vi "Handle Command.vi"(8 "error in (no error)":errorcluster, 9 "Data":variant, 10 "Command":string, 11 "Instrument.Oxford1820 in":refnum<class "Instrument.OxfordVRM.lvclass">) -> (0 "error out":errorcluster, 1 "Processed Data":variant, 2 "Command":string, 3 "Instrument.Oxford1820 out":refnum<class "Instrument.OxfordVRM.lvclass">)   [LabVIEW 2016, in "Instrument.OxfordVRM.lvclass"]
uses:
  Instrument.OxfordVRM.lvclass
  Typedefs/Instrument.Oxford1820.Commands-enum.ctl
  <instrlib>/Mercury iXX/Public/Libraries/Magnet/Controls/PSU Actions.ctl
  Typedefs/Targets.ctl
  Typedefs/PrivateEvents--Instrument.Oxford1820.SequenceSetMagnetField.ctl
  Typedefs/Instrument.Oxford1820.setMagnet-cluster.ctl
  <instrlib>/Mercury iXX/Public/Libraries/Magnet/Controls/Switch Heater.ctl
  Typedefs/Fill Mode-Combo.ctl
  <userlib>/LevyLab/Levylab Instruments/Instrument Types/Cryostat/Instrument.Cryostat.lvclass
  <instrlib>/Mercury iXX/Public/Libraries/Magnet.lvlib
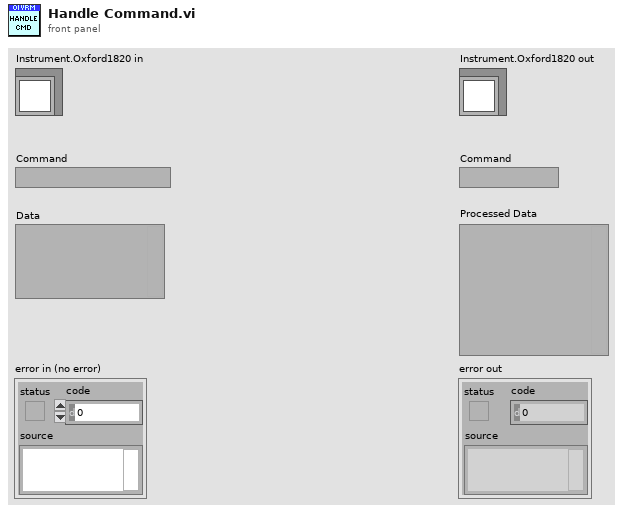
[diagram p1: front panel]
types:
  T1 = typedef "Instrument.OxfordVRM.lvclass/Instrument.Oxford1820.Commands-enum.ctl" = enum16{"setAction", "setTarget", "setSwitchHeat", "setLambda", "setFillMode", "setNeedleValve", "setMagnetField", "getStatus", "getTarget", "getSwitchHeat", "getPSUField", "newcommand", "getMagnetField"}
  T2 = typedef "Mercury iXX.lvlib/Magnet.lvlib/PSU Actions.ctl" = string
  T3 = typedef "Instrument.OxfordVRM.lvclass/Targets.ctl" = cluster{"Field (T)":dbl, "Field Rate (T/min)":dbl}
  T4 = typedef "Instrument.OxfordVRM.lvclass/Instrument.Oxford1820.setMagnet-cluster.ctl" = cluster{"Target":T3, "persistent mode":bool}
  T5 = typedef "Instrument.OxfordVRM.lvclass/PrivateEvents--Instrument.Oxford1820.SequenceSetMagnetField.ctl" = cluster{"setMagnet":T4}
  T6 = typedef "Mercury iXX.lvlib/Magnet.lvlib/Switch Heater.ctl" = string
  T7 = typedef "Instrument.OxfordVRM.lvclass/Fill Mode-Combo.ctl" = string
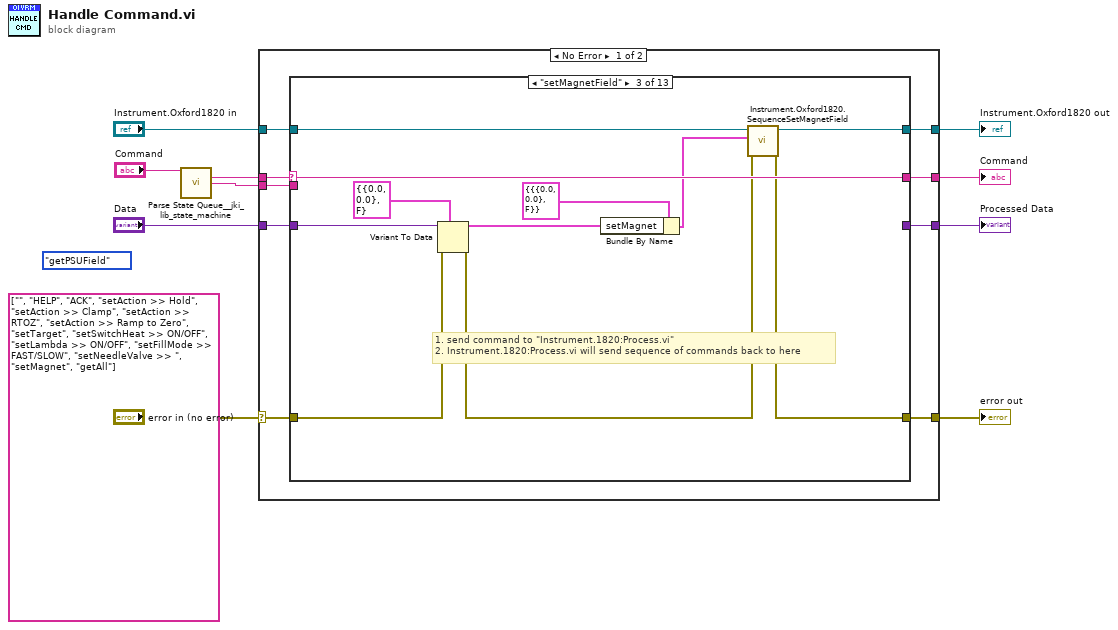
[diagram p0: block diagram]
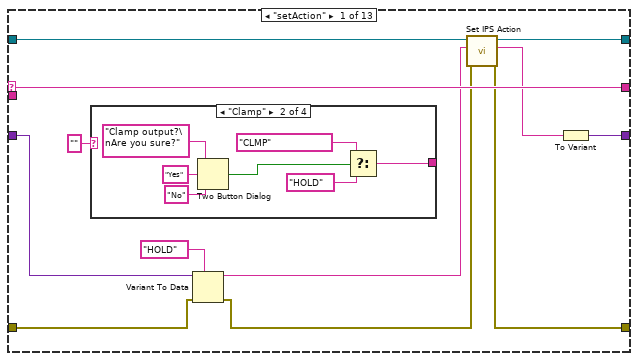
[diagram p2: hidden frame]
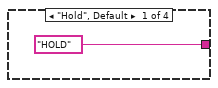
[diagram p3: hidden frame]
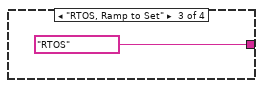
[diagram p4: hidden frame]
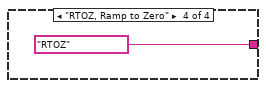
[diagram p5: hidden frame]
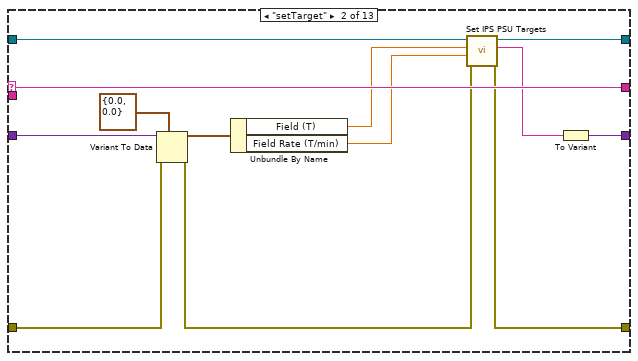
[diagram p6: hidden frame]
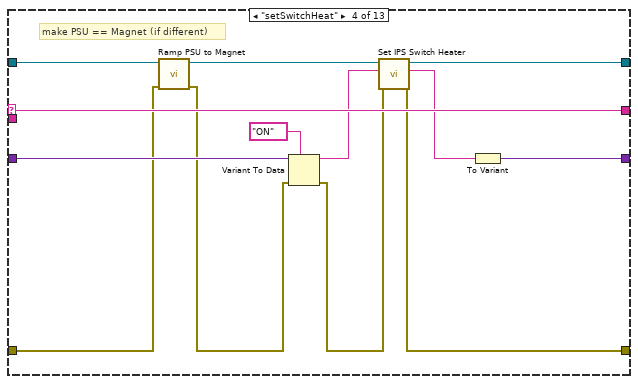
[diagram p7: hidden frame]
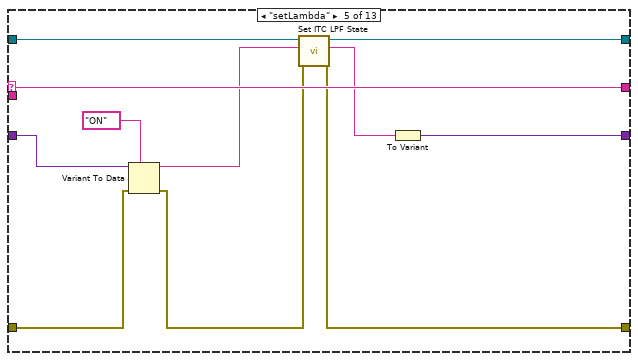
[diagram p8: hidden frame]
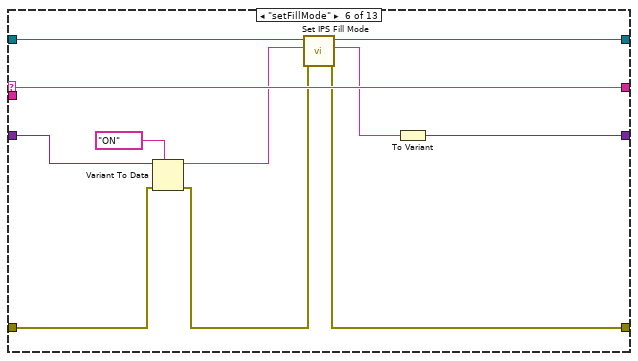
[diagram p9: hidden frame]
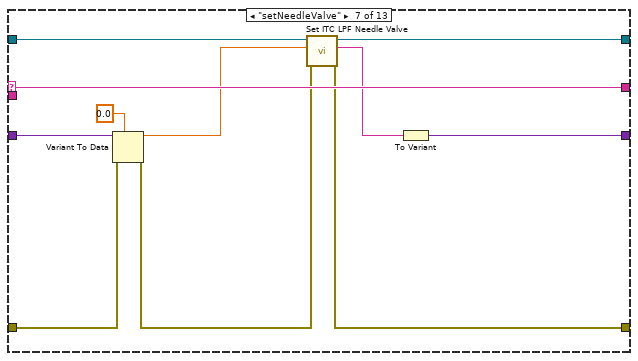
[diagram p10: hidden frame]
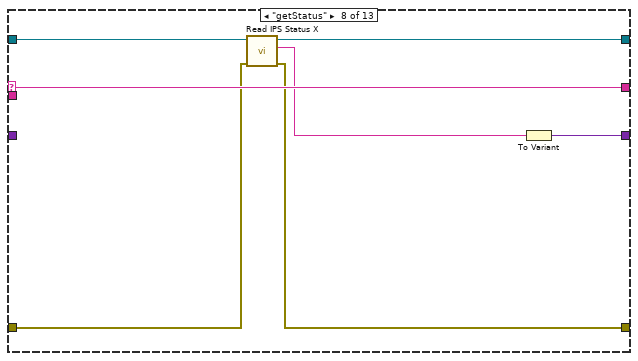
[diagram p11: hidden frame]
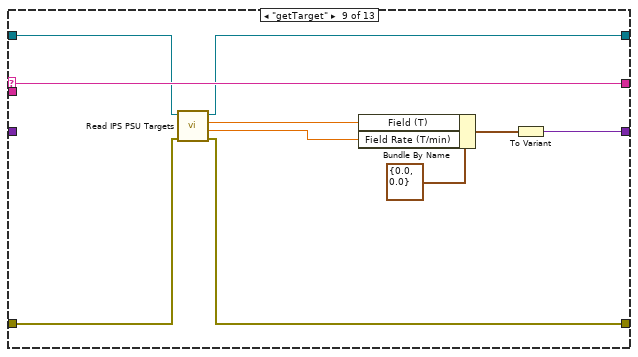
[diagram p12: hidden frame]
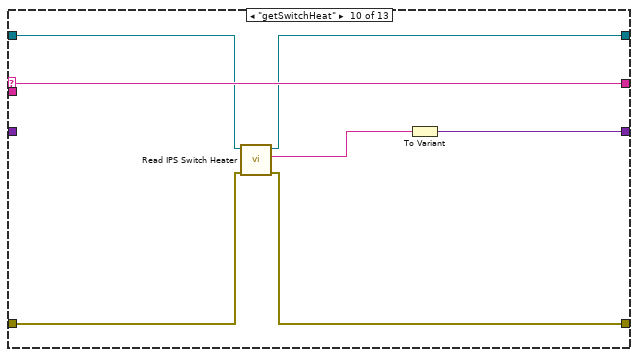
[diagram p13: hidden frame]
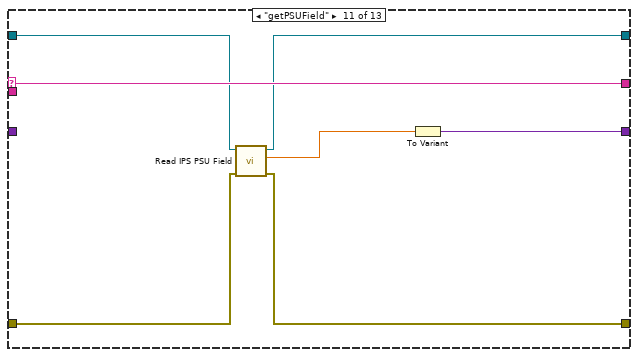
[diagram p14: hidden frame]
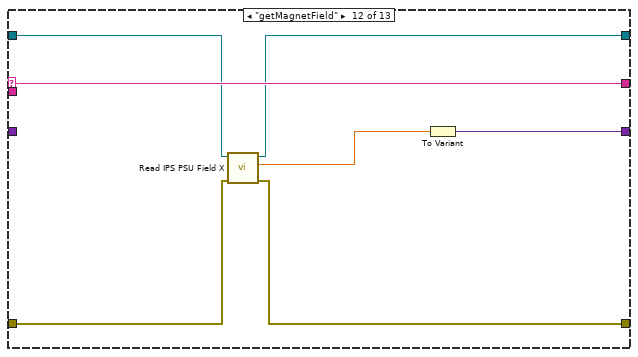
[diagram p15: hidden frame]
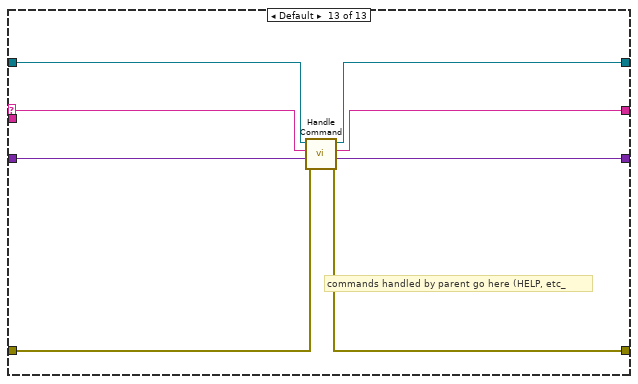
[diagram p16: hidden frame]
diagram:
  (unwired) Instrument.Oxford1820.Commands-enum."getPSUField" ("Commands")
  (unwired) string[] ["", "HELP", "ACK", "setAction >> Hold", "setAction >> Clamp", "setAction >> RTOZ", "setAction >> Ramp to Zero", "setTarget", "setSwitchHeat >> ON/OFF", "setLambda >> ON/OFF", "setFillMode >> FAST/SLOW", "setNeedleValve >> ", "setMagnet", "getAll"] ("Commands")
  n1 = call <vilib>:"Parse State Queue__jki_lib_state_machine.vi"("State Queue"="Command") -> ("Current State"=w2:string, "Arguments"=w1:string)  [unwired: 12 in, 1 out]
  n2 = case shown="No Error" "error in (no error)" {
    selector: "error in (no error)" -> [w14 w158]
    tunnel: [w13 w158] -> w10
    tunnel: [w19 _] -> w9
    tunnel: [w18 _] -> w8
    tunnel: [w17 w159] -> w7
    tunnel: "Data" -> [w16 _]
    tunnel: w2 -> [w11 _]
    tunnel: "Instrument.Oxford1820 in" -> [w15 w159]
    tunnel: w1 -> [w12 _]
    frame No Error {
      n3 = case shown="\"setMagnetField\"" w11 {
        selector: w11 -> [w31 w54 w65 w78 w89 w100 w111 w118 w128 w135 w142 w149 w150]
        tunnel: [w26 w49 _ w74 w84 w95 w106 w117 w127 w134 w141 w148 w157] -> w19
        tunnel: [w31 w54 w65 w78 w89 w100 w111 w118 w128 w135 w142 w149 w156] -> w18
        tunnel: [w29 w52 w63 w77 w87 w98 w109 w112 w120 w132 w139 w147 w155] -> w17
        tunnel: w16 -> [w25 w48 w61 w71 w82 w94 w104 _ _ _ _ _ w154]
        tunnel: w15 -> [w30 w53 w64 w73 w88 w99 w110 w113 w119 w133 w140 w143 w153]
        tunnel: w14 -> [w23 w43 w60 w69 w81 w92 w102 w116 w122 w131 w138 w145 w152]
        tunnel: [w28 w51 w62 w76 w86 w97 w108 w115 w121 w130 w137 w144 w151] -> w13
        tunnel: w12 -> [_ _ _ _ _ _ _ _ _ _ _ _ _]
        frame "setAction" {
          n4 = case shown="\"Clamp\"" "" {
            tunnel: [T2 "HOLD" ("PSU Act Stat") w38 T2 "RTOS" ("PSU Act Stat") T2 "RTOZ" ("PSU Act Stat")] -> _
            frame "Hold", Default {
            }
            frame "Clamp" {
              n5 = Two Button Dialog(message="Clamp output?\nAre you sure?", 1:"No" ("F button name (\"Cancel\")"), 2:"Yes" ("T button name (\"OK\")")) -> (T button?=w37:bool)
              n6 = Select(t=T2 "CLMP" ("PSU Act Stat"), s=w37, f=T2 "HOLD" ("PSU Act Stat")) -> (s? t:f=w38:T2)
            }
            frame "RTOS, Ramp to Set" {
            }
            frame "RTOZ, Ramp to Zero" {
            }
          }
          n7 = Variant To Data(error in=w23, type=T2 "HOLD" ("PSU Act Stat"), Variant=w25) -> (data=w21:T2, error out=w22:errorcluster)
          n8 = call "Set IPS Action.vi"("error in (no error)"=w22, "PSU Act Stat"=w21, "Instrument.OxfordVRM in"=w30) -> ("error out"=w28:errorcluster, "Response"=w27:string, "Instrument.OxfordVRM out"=w29:refnum<class "Instrument.OxfordVRM.lvclass">)  [unwired: 6 in]
          n9 = To Variant(anything=w27) -> (Variant=w26:variant)
        }
        frame "setTarget" {
          n10 = Variant To Data(error in=w43, type=T3 {"Field (T)"=0.0, "Field Rate (T/min)"=0.0} ("Targets"), Variant=w48) -> (data=w46:T3, error out=w42:errorcluster)
          n11 = Unbundle By Name(w46) -> ("Field (T)"=w45:dbl, "Field Rate (T/min)"=w44:dbl)
          n12 = call "Set IPS PSU Targets.vi"("error in (no error)"=w42, "Target Field Rate (T/min)"=w44, "Target Field (T)"=w45, "Instrument.OxfordVRM in"=w53) -> ("error out"=w51:errorcluster, "Response"=w50:string, "Instrument.OxfordVRM out"=w52:refnum<class "Instrument.OxfordVRM.lvclass">)  [unwired: 5 in]
          n13 = To Variant(anything=w50) -> (Variant=w49:variant)
        }
        frame "setMagnetField" {
          # "1. send command to \"Instrument.1820:Process.vi\"\n2. Instrument.1820:Process.vi will send sequence of commands back to here"
          n14 = Variant To Data(error in=w60, type=T4 {"Target"={"Field (T)"=0.0, "Field Rate (T/min)"=0.0}, "persistent mode"=FALSE} ("output cluster"), Variant=w61) -> (data=w56:T4, error out=w59:errorcluster)
          n15 = Bundle By Name(cluster=T5 {"setMagnet"={"Target"={"Field (T)"=0.0, "Field Rate (T/min)"=0.0}, "persistent mode"=FALSE}} ("Set Magnet Field"), "setMagnet"=w56) -> (w58:T5)
          n16 = call "Instrument.Oxford1820.SequenceSetMagnetField.vi"("error in (no error)"=w59, "Set Magnet Field"=w58, "Instrument.Oxford1820"=w64) -> ("error out"=w62:errorcluster, "Instrument.Oxford1820 out"=w63:refnum<class "Instrument.OxfordVRM.lvclass">)  [unwired: 7 in]
        }
        frame "setSwitchHeat" {
          # "make PSU == Magnet (if different)"
          n17 = call "Ramp PSU to Magnet.vi"("error in (no error)"=w69, "Instrument.VRM in"=w73) -> ("error out"=w68:errorcluster, "Instrument.VRM out"=w72:refnum<class "Instrument.OxfordVRM.lvclass">)  [unwired: 8 in]
          n18 = Variant To Data(error in=w68, type=T6 "ON" ("Switch Heater Status"), Variant=w71) -> (data=w70:T6, error out=w67:errorcluster)
          n19 = call "Set IPS Switch Heater.vi"("error in (no error)"=w67, "Switch Heater Status"=w70, "Instrument.Oxford1820 in"=w72) -> ("error out"=w76:errorcluster, "Response"=w75:string, "Instrument.Oxford1820 out"=w77:refnum<class "Instrument.OxfordVRM.lvclass">)  [unwired: 6 in]
          n20 = To Variant(anything=w75) -> (Variant=w74:variant)
        }
        frame "setLambda" {
          n21 = Variant To Data(error in=w81, type=T6 "ON" ("LPF State"), Variant=w82) -> (data=w80:T6, error out=w79:errorcluster)
          n22 = call "Set ITC LPF State.vi"("error in (no error)"=w79, "LPF State"=w80, "Instrument.Oxford1820 in"=w88) -> ("error out"=w86:errorcluster, "Response"=w85:string, "Instrument.Oxford1820 out"=w87:refnum<class "Instrument.OxfordVRM.lvclass">)  [unwired: 6 in]
          n23 = To Variant(anything=w85) -> (Variant=w84:variant)
        }
        frame "setFillMode" {
          n24 = Variant To Data(error in=w92, type=T7 "ON" ("Fill Mode"), Variant=w94) -> (data=w90:T7, error out=w91:errorcluster)
          n25 = call "Set IPS Fill Mode.vi"("error in (no error)"=w91, "Fill Mode"=w90, "Instrument.Oxford1820 in"=w99) -> ("error out"=w97:errorcluster, "Response"=w96:string, "Instrument.Oxford1820 out"=w98:refnum<class "Instrument.OxfordVRM.lvclass">)  [unwired: 6 in]
          n26 = To Variant(anything=w96) -> (Variant=w95:variant)
        }
        frame "setNeedleValve" {
          n27 = Variant To Data(error in=w102, type=0.0 ("Percentage Open (%)"), Variant=w104) -> (data=w103:dbl, error out=w101:errorcluster)
          n28 = call "Set ITC LPF Needle Valve.vi"("error in (no error)"=w101, "Percentage Open (%)"=w103, "Instrument.Oxford1820 in"=w110) -> ("error out"=w108:errorcluster, "Response"=w107:string, "Instrument.Oxford1820 out"=w109:refnum<class "Instrument.OxfordVRM.lvclass">)  [unwired: 6 in]
          n29 = To Variant(anything=w107) -> (Variant=w106:variant)
        }
        frame "getStatus" {
          n30 = call "Read IPS Status X.vi"("error in (no error)"=w116, "Instrument.OxfordVRM in"=w113) -> ("error out"=w115:errorcluster, "Status"=w114:string, "Instrument.OxfordVRM out"=w112:refnum<class "Instrument.OxfordVRM.lvclass">)  [unwired: 7 in]
          n31 = To Variant(anything=w114) -> (Variant=w117:variant)
        }
        frame "getTarget" {
          n32 = call "Read IPS PSU Targets.vi"("error in (no error)"=w122, "Instrument.OxfordVRM in"=w119) -> ("error out"=w121:errorcluster, "Target Field Rate (T/min)"=w123:dbl, "Target Field (T)"=w124:dbl, "Instrument.OxfordVRM out"=w120:refnum<class "Instrument.OxfordVRM.lvclass">)  [unwired: 6 in]
          n33 = Bundle By Name(cluster=T3 {"Field (T)"=0.0, "Field Rate (T/min)"=0.0} ("Target"), "Field (T)"=w124, "Field Rate (T/min)"=w123) -> (w126:T3)
          n34 = To Variant(anything=w126) -> (Variant=w127:variant)
        }
        frame "getSwitchHeat" {
          n35 = call "Read IPS Switch Heater.vi"("error in (no error)"=w131, "Instrument.Oxford1820 in"=w133) -> ("error out"=w130:errorcluster, "Switch Heater Status"=w129:string, "Instrument.Oxford1820 out"=w132:refnum<class "Instrument.OxfordVRM.lvclass">)  [unwired: 6 in, 1 out]
          n36 = To Variant(anything=w129) -> (Variant=w134:variant)
        }
        frame "getPSUField" {
          n37 = call "Read IPS PSU Field.vi"("error in (no error)"=w138, "Instrument.OxfordVRM in"=w140) -> ("error out"=w137:errorcluster, "Power Supply Field (T)"=w136:dbl, "Instrument.OxfordVRM out"=w139:refnum<class "Instrument.OxfordVRM.lvclass">)  [unwired: 7 in]
          n38 = To Variant(anything=w136) -> (Variant=w141:variant)
        }
        frame "getMagnetField" {
          n39 = call "Read IPS PSU Field X.vi"("error in (no error)"=w145, "Instrument.OxfordVRM in"=w143) -> ("error out"=w144:errorcluster, "Magnet Field (T)"=w146:dbl, "Instrument.OxfordVRM out"=w147:refnum<class "Instrument.OxfordVRM.lvclass">)  [unwired: 7 in]
          n40 = To Variant(anything=w146) -> (Variant=w148:variant)
        }
        frame Default {
          # "commands handled by parent go here (HELP, etc_"
          n41 = call-parent "Handle Command.vi"("error in (no error)"=w152, "Data"=w154, "Command"=w150, "Instrument in"=w153) -> ("error out"=w151:errorcluster, "Processed Data"=w157:variant, "Command"=w156:string, "Instrument out"=w155:refnum<class "Instrument.OxfordVRM.lvclass">)  [unwired: 4 in]
        }
      }
    }
    frame Error {
    }
  }
  "error out" <- w10
  "Instrument.Oxford1820 out" <- w7
  "Processed Data" <- w9
  "Command" <- w8
